vi "HT_Contents_IMAQDevice.vi"   [LabVIEW 2014]
doc: "This \"contents\" VI contains all components of CS, which are specific for YOU, a CS user. Add your own stuff here."
uses:
  CSVision/IMAQDevice/IMAQDevice.lvlib
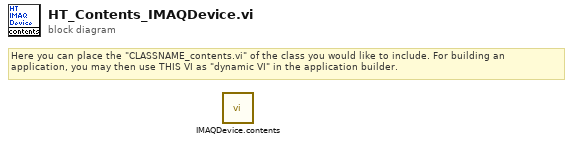
[diagram p0: block diagram]
diagram:
  # "Here you can place the \"CLASSNAME_contents.vi\" of the class you would like to include. For building an \napplication, you may then use THIS VI as \"dynamic VI\" in the application builder."
  n1 = call "IMAQDevice.contents.vi"() -> ()  [unwired: 1 in]
